vi "Return All Four Axis Positions.vi"(8 "error in (no error)":errorcluster, 11 "VISA resource name":refnum<visa-resource-name>) -> (0 "error out":errorcluster, 1 "Positions, counts":i32[](array[numeric]), 3 "VISA resource out":refnum<visa-resource-name>)   [LabVIEW 2017]
doc: "Read all four positions.\nCannot be used while in motion, only when VXM status is R"
panel:
  out "i":i32
  out "Strings":string[](array[string])
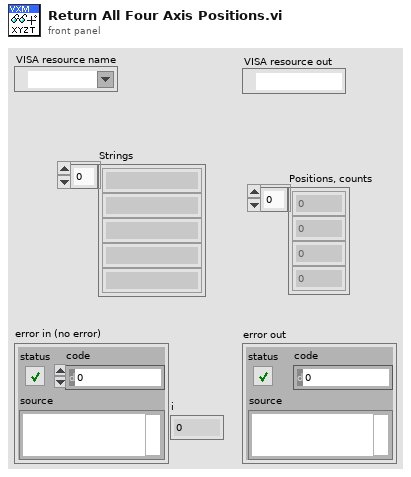
[diagram p1: front panel]
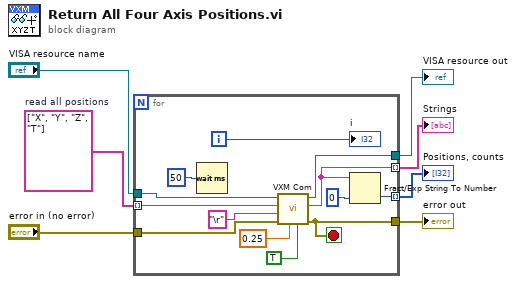
[diagram p0: block diagram]
diagram:
  w7 = string[] ["X", "Y", "Z", "T"]  # read all positions
  n1 = for {
    tunnel: [w18] -> w2 mode=indexing
    tunnel: w7 -> [w17] mode=indexing
    tunnel: "VISA resource name" -> [w16]
    tunnel: [w15] -> w5
    tunnel: [w13] -> w4
    tunnel: "error in (no error)" -> [w14]
    tunnel: [w9] -> w1 mode=indexing
    i -> [w10]
    stop <- w13 stop-if-true
    n2 = Wait (ms)(milliseconds to wait=u32 50) -> ()  [unwired: 1 out]
    n3 = call "VXM Com.vi"("Flush RS232"=TRUE, "Timeout, s"=0.25, "error in (no error)"=w14, "Termination String ('/' codes)"="\r", "Write Buffer ('/' codes)"=w17, "VISA resource name"=w16) -> ("error out"=w13:errorcluster, "Response String ('/' codes)"=w9:string, "VISA resource out"=w15:refnum<visa-resource-name>)  [unwired: 3 in]
    n4 = Fract/Exp String To Number(string=w9, default (0 dbl)=0 ("default (0 DBL)")) -> (number=w18:i32)  [unwired: 2 in, 1 out]
    "i" <- w10
  }
  "VISA resource out" <- w5
  "error out" <- w4
  "Positions, counts" <- w2
  "Strings" <- w1
